vi "GenerateMatchingWave.vi"(6 "Num of Waves":dbl=1.0, 8 "Frequency":dbl=1.0, 9 "phase in":dbl format="%0.2f", 10 "Offset":dbl=50.0, 11 "Amplitude":dbl=50.0) -> (3 "Gait 2":cluster{i32, dbl}[](graph), 4 "X Scale":i32[](array[numeric]))   [LabVIEW 2011]
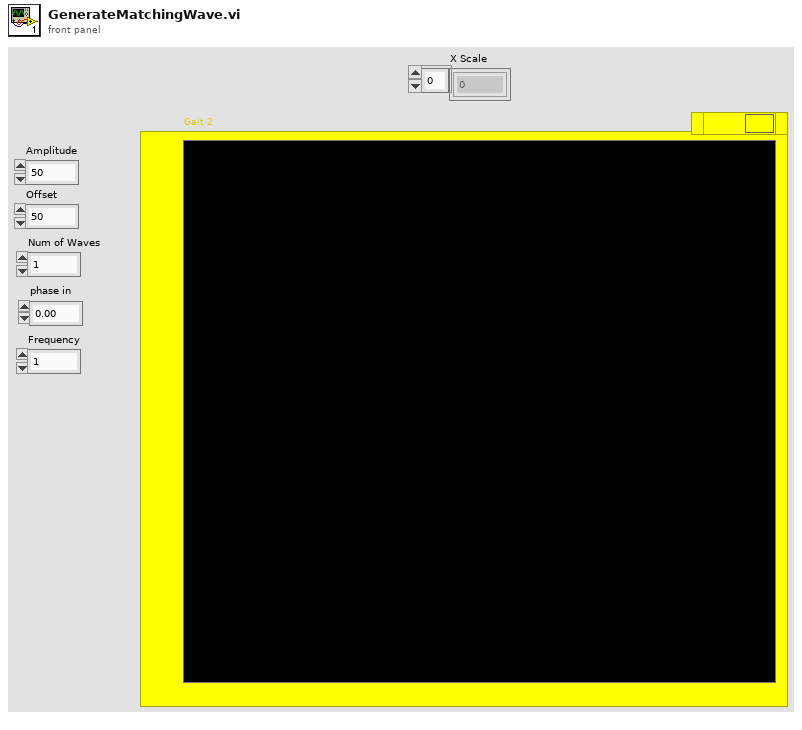
[diagram p1: front panel]
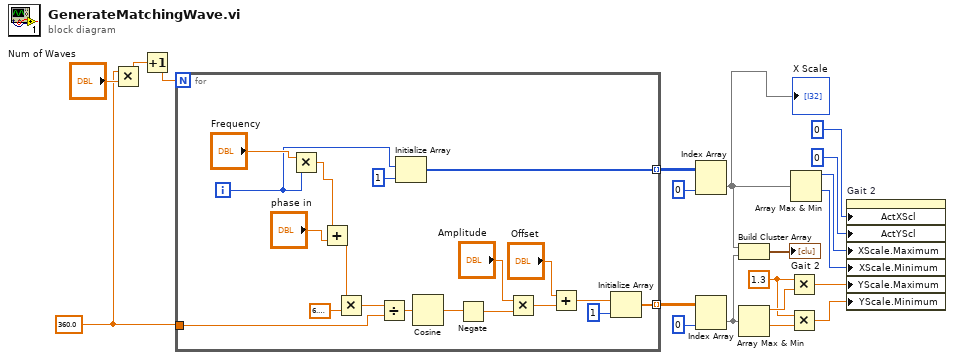
[diagram p0: block diagram]
diagram:
  w6 = 1.3 ("x")
  w19 = 360.0 ("x")
  n1 = Multiply(x=w19, y="Num of Waves") -> (x*y=w4:dbl)
  n2 = Increment(x=w4) -> (x+1=w3:dbl)
  n3 = for {
    N: w3 -> [_]
    tunnel: [w39] -> w17 mode=indexing
    tunnel: w19 -> [w35]
    tunnel: [w32] -> w18 mode=indexing
    i -> [w22]
    n4 = Multiply(x="Frequency", y=w22) -> (x*y=w21:dbl)
    n5 = Add(x=w21, y="phase in") -> (x+y=w24:dbl)
    n6 = Multiply(x=w24, y=6.283185307179586) -> (x*y=w36:dbl)
    n7 = Divide(x=w36, y=w35) -> (x/y=w34:dbl)
    n8 = Initialize Array(w22, 1 ("dimension size")) -> (w32:i32[])
    n9 = Cosine(x=w34) -> (cos(x)=w27:dbl)
    n10 = Negate(x=w27) -> (-x=w26:dbl)
    n11 = Multiply(x="Amplitude", y=w26) -> (x*y=w30:dbl)
    n12 = Add(x="Offset", y=w30) -> (x+y=w29:dbl)
    n13 = Initialize Array(w29, 1 ("dimension size")) -> (w39:dbl[])
  }
  n14 = Index Array(array=w18, index (col)=0 ("index (row)")) -> (element=w2:i32[])  [unwired: 1 in]
  "X Scale" <- w2
  n15 = Index Array(array=w17, index (col)=0 ("index (row)")) -> (element=w1:dbl[])  [unwired: 1 in]
  n16 = Build Cluster Array ("Index & Bundle Cluster Array")(w2, w1) -> (→"Gait 2":cluster{i32, dbl}[])
  n17 = Array Max & Min(array=w1) -> (max value=w9:dbl, min value=w7:dbl)  [unwired: 2 out]
  n18 = Multiply(x=w6, y=w9) -> (x*y=w8:dbl)
  n19 = Multiply(x=w6, y=w7) -> (x*y=w5:dbl)
  n20 = Array Max & Min(array=w2) -> (max value=w13:i32, min value=w12:i32)  [unwired: 2 out]
  n21 = property on="Gait 2" class="XYGraph (strict)"("ActXScl"=0 ("Active X Scale"), "ActYScl"=0 ("Active Y Scale"), "XScale.Maximum"=w13, "XScale.Minimum"=w12, "YScale.Maximum"=w8, "YScale.Minimum"=w5) -> ()  [unwired: 2 in, 2 out]
